vi "_Process Old Elements.vi"(8 "Input Text":string) -> (0 "error out":errorcluster, 1 "Processed Text":string)   [LabVIEW 2012]
panel:
  in  "HTML File Path":path
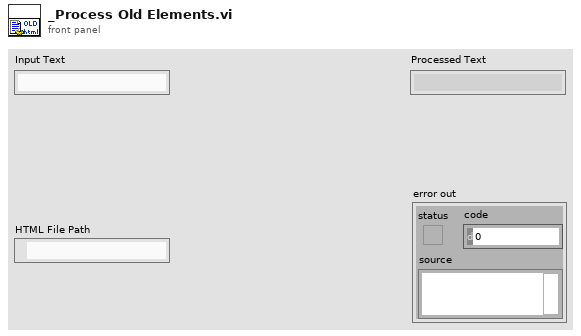
[diagram p1: front panel]
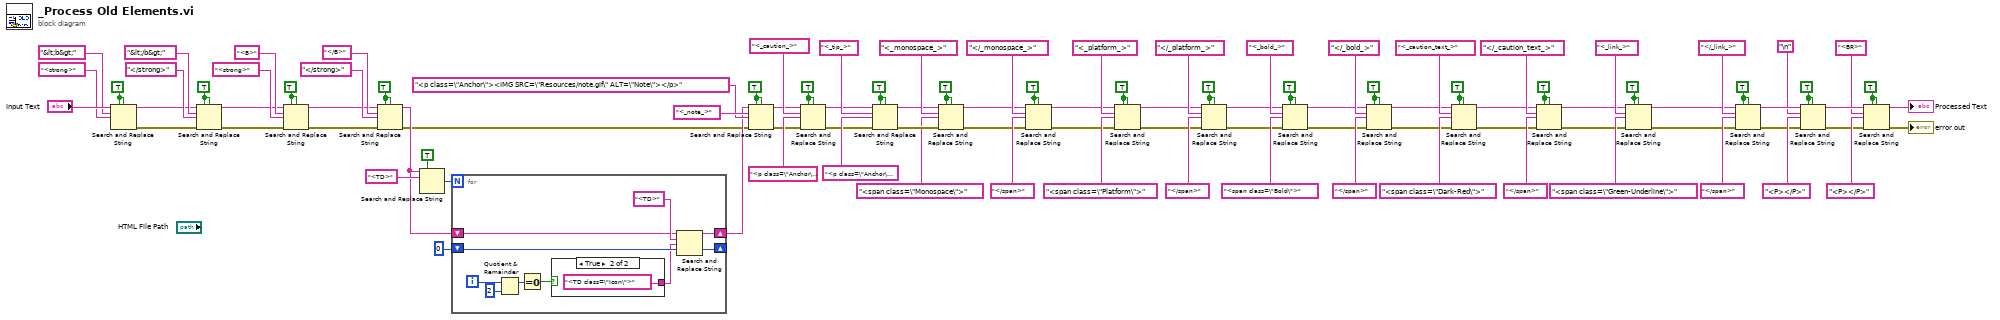
[diagram p0: block diagram]
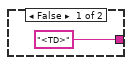
[diagram p2: hidden frame]
diagram:
  w7 = TRUE ("replace all? (F)")
  w12 = TRUE ("replace all? (F)")
  w18 = TRUE ("replace all? (F)")
  w21 = TRUE ("replace all? (F)")
  w28 = TRUE ("replace all? (F)")
  w31 = TRUE ("replace all? (F)")
  w38 = TRUE ("replace all? (F)")
  w41 = TRUE ("replace all? (F)")
  w48 = TRUE ("replace all? (F)")
  w51 = TRUE ("replace all? (F)")
  w56 = TRUE ("replace all? (F)")
  w61 = TRUE ("replace all? (F)")
  w67 = TRUE ("replace all? (F)")
  w70 = TRUE ("replace all? (F)")
  w75 = TRUE ("replace all? (F)")
  w78 = TRUE ("replace all? (F)")
  w79 = TRUE ("replace all? (F)")
  w80 = TRUE ("replace all? (F)")
  w81 = TRUE ("replace all? (F)")
  n1 = Search and Replace String(replace all?=w81, case sensitive?=w81, input string="Input Text", search string="&lt;b&gt;", replace string="<strong>" ("replace string (\"\")")) -> (result string=w95:string, error out=w96:errorcluster)  [unwired: 3 in, 2 out]
  n2 = Search and Replace String(replace all?=w80, case sensitive?=w80, input string=w95, search string="&lt;/b&gt;", replace string="</strong>" ("replace string (\"\")"), error in=w96) -> (result string=w87:string, error out=w88:errorcluster)  [unwired: 2 in, 2 out]
  n3 = Search and Replace String(replace all?=w79, case sensitive?=w79, input string=w87, search string="<B>", replace string="<strong>" ("replace string (\"\")"), error in=w88) -> (result string=w89:string, error out=w90:errorcluster)  [unwired: 2 in, 2 out]
  n4 = Search and Replace String(replace all?=w78, case sensitive?=w78, input string=w89, search string="</B>", replace string="</strong>" ("replace string (\"\")"), error in=w90) -> (result string=w83:string, error out=w73:errorcluster)  [unwired: 2 in, 2 out]
  n5 = Search and Replace String(replace all?=TRUE ("replace all? (F)"), input string=w83, search string="<TD>") -> (number of replacements=w84:i32)  [unwired: 5 in, 3 out]
  n6 = for {
    N: w84 -> [_]
    shift-right: [w107] -> w74
    shift-left: w83 -> [w104]
    shift-right: [w106] -> _
    shift-left: 0 -> [w103]
    i -> [w111]
    n7 = Quotient & Remainder(x=w111, y=2) -> (x-y*floor(x/y)=w109:i32)  [unwired: 1 out]
    n8 = Equal To 0?(x=w109) -> (x = 0?=w108:bool)
    n9 = case shown="True" w108 {
      tunnel: ["<TD>" ("search string") "<TD class=\"Icon\">" ("replace string (\"\")")] -> w102
      frame False {
      }
      frame True {
      }
    }
    n10 = Search and Replace String(input string=w104, search string="<TD>", replace string=w102, offset=w103) -> (result string=w107:string, offset past replacement=w106:i32)  [unwired: 4 in, 2 out]
  }
  n11 = Search and Replace String(replace all?=w75, case sensitive?=w75, input string=w74, search string="<_note_>", replace string="<p class=\"Anchor\"><IMG SRC=\"Resources/note.gif\" ALT=\"Note\"></p>" ("replace string (\"\")"), error in=w73) -> (result string=w66:string, error out=w65:errorcluster)  [unwired: 2 in, 2 out]
  n12 = Search and Replace String(replace all?=w70, case sensitive?=w70, input string=w66, search string="<_caution_>", replace string="<p class=\"Anchor\"><IMG SRC=\"Resources/caution.gif\" ALT=\"Caution\"></p>" ("replace string (\"\")"), error in=w65) -> (result string=w63:string, error out=w64:errorcluster)  [unwired: 2 in, 2 out]
  n13 = Search and Replace String(replace all?=w67, case sensitive?=w67, input string=w63, search string="<_tip_>", replace string="<p class=\"Anchor\"><IMG SRC=\"Resources/tip.gif\" ALT=\"Tip\"></p>" ("replace string (\"\")"), error in=w64) -> (result string=w59:string, error out=w60:errorcluster)  [unwired: 2 in, 2 out]
  n14 = Search and Replace String(replace all?=w61, case sensitive?=w61, input string=w59, search string="<_monospace_>", replace string="<span class=\"Monospace\">", error in=w60) -> (result string=w53:string, error out=w54:errorcluster)  [unwired: 2 in, 2 out]
  n15 = Search and Replace String(replace all?=w56, case sensitive?=w56, input string=w53, search string="</_monospace_>", replace string="</span>", error in=w54) -> (result string=w43:string, error out=w44:errorcluster)  [unwired: 2 in, 2 out]
  n16 = Search and Replace String(replace all?=w51, case sensitive?=w51, input string=w43, search string="<_platform_>", replace string="<span class=\"Platform\">", error in=w44) -> (result string=w45:string, error out=w46:errorcluster)  [unwired: 2 in, 2 out]
  n17 = Search and Replace String(replace all?=w48, case sensitive?=w48, input string=w45, search string="</_platform_>", replace string="</span>", error in=w46) -> (result string=w33:string, error out=w34:errorcluster)  [unwired: 2 in, 2 out]
  n18 = Search and Replace String(replace all?=w41, case sensitive?=w41, input string=w33, search string="<_bold_>", replace string="<span class=\"Bold\">", error in=w34) -> (result string=w35:string, error out=w36:errorcluster)  [unwired: 2 in, 2 out]
  n19 = Search and Replace String(replace all?=w38, case sensitive?=w38, input string=w35, search string="</_bold_>", replace string="</span>", error in=w36) -> (result string=w23:string, error out=w24:errorcluster)  [unwired: 2 in, 2 out]
  n20 = Search and Replace String(replace all?=w31, case sensitive?=w31, input string=w23, search string="<_caution_text_>", replace string="<span class=\"Dark-Red\">", error in=w24) -> (result string=w25:string, error out=w26:errorcluster)  [unwired: 2 in, 2 out]
  n21 = Search and Replace String(replace all?=w28, case sensitive?=w28, input string=w25, search string="</_caution_text_>", replace string="</span>", error in=w26) -> (result string=w13:string, error out=w14:errorcluster)  [unwired: 2 in, 2 out]
  n22 = Search and Replace String(replace all?=w21, case sensitive?=w21, input string=w13, search string="<_link_>", replace string="<span class=\"Green-Underline\">", error in=w14) -> (result string=w15:string, error out=w16:errorcluster)  [unwired: 2 in, 2 out]
  n23 = Search and Replace String(replace all?=w18, case sensitive?=w18, input string=w15, search string="</_link_>", replace string="</span>", error in=w16) -> (result string=w9:string, error out=w10:errorcluster)  [unwired: 2 in, 2 out]
  n24 = Search and Replace String(replace all?=w12, case sensitive?=w12, input string=w9, search string="\n", replace string="<P></P>", error in=w10) -> (result string=w4:string, error out=w5:errorcluster)  [unwired: 2 in, 2 out]
  n25 = Search and Replace String(replace all?=w7, case sensitive?=w7, input string=w4, search string="<BR>", replace string="<P></P>", error in=w5) -> (result string=→"Processed Text":string, error out=→"error out":errorcluster)  [unwired: 2 in, 2 out]
